vi "GetRecord.vi"(8 "error in (no error)":errorcluster, 10 "Label":string, 11 "Task_Abstr in":refnum<class "Task_Abstr.lvclass">) -> (0 "error out":errorcluster, 2 "WaveformData":T1 {"StopTime" format="%<%x %.3X>T"; "StartTime" format="%<%x %.3X>T"}, 3 "Task_Abstr out":refnum<class "Task_Abstr.lvclass">)   [LabVIEW 2025, in "Task_Abstr.lvlib" / "Task_Abstr.lvclass"]
uses:
  Task_Abstr.lvclass
  WaveformData.ctl
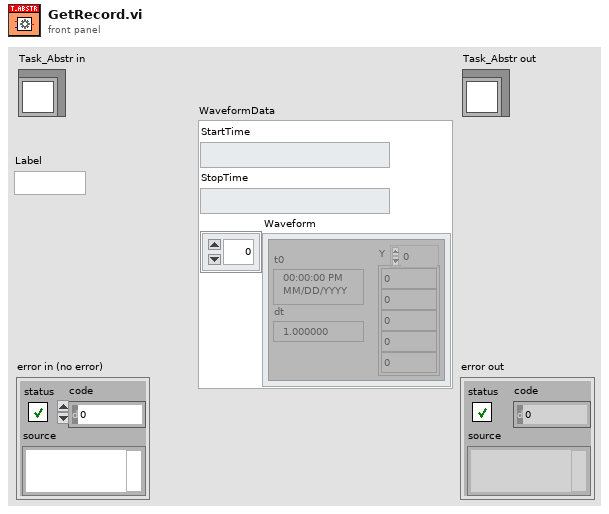
[diagram p1: front panel]
types:
  T1 = typedef "Task_Abstr.lvlib/Task_Abstr.lvclass/WaveformData.ctl" = cluster{"StartTime":timestamp, "StopTime":timestamp, "Waveform":waveform(dbl)[]}
  T2 = typedef "Task_Abstr.lvlib/Task_Abstr.lvclass/DataContainer.ctl" = map{string, T1}
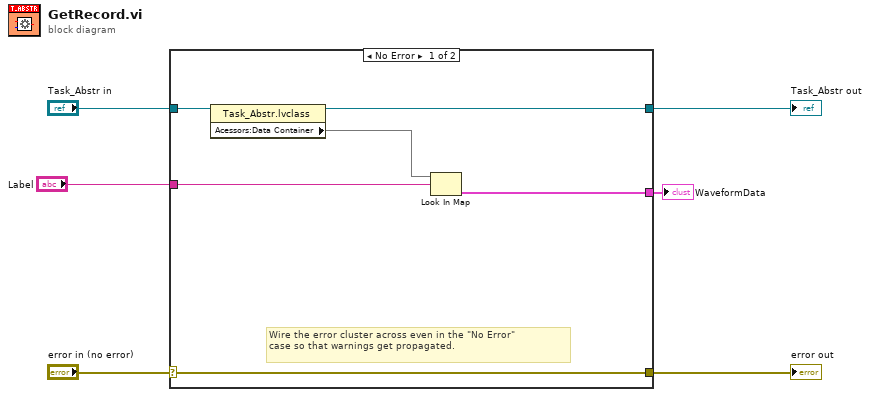
[diagram p0: block diagram]
diagram:
  n1 = case shown="No Error" "error in (no error)" {
    selector: "error in (no error)" -> [w11 w14]
    tunnel: [w11 w14] -> w5
    tunnel: [w10 w13] -> w3
    tunnel: "Task_Abstr in" -> [w12 w13]
    tunnel: "Label" -> [w8 _]
    tunnel: [w7 _] -> w1
    frame No Error {
      # "Wire the error cluster across even in the \"No Error\"\ncase so that warnings get propagated."
      n2 = property class="Task_Abstr.lvclass"(reference=w12) -> (reference out=w10:refnum<class "Task_Abstr.lvclass">, "Acessors:Data Container"=w9:T2)  [unwired: 1 in, 1 out]
      n3 = Look In Map(map=w9, key=w8) -> (value=w7:T1)  [unwired: 1 in, 1 out]
    }
    frame Error {
    }
  }
  "error out" <- w5
  "Task_Abstr out" <- w3
  "WaveformData" <- w1
